vi "parse_add_vector_response.vi"(0 "headers":string, 5 "body":string, 11 "error in (no error)":errorcluster) -> (15 "error out":errorcluster)   [LabVIEW 2020, in "vector_weviate.lvclass"]
doc: "This VI parses the response of the Add Vector request"
uses:
  vector_weviate.lvclass
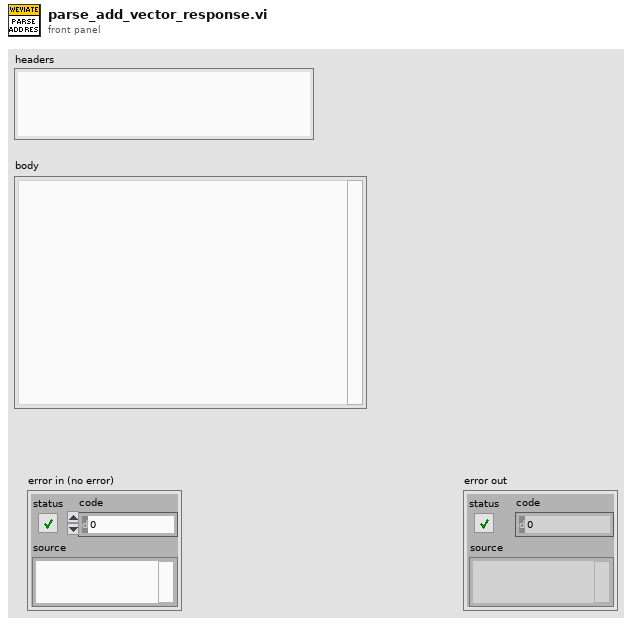
[diagram p1: front panel]
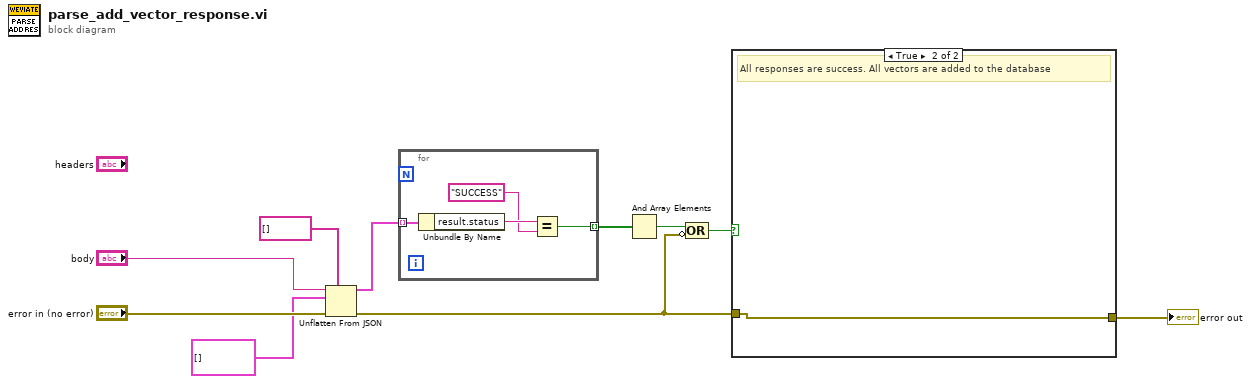
[diagram p0: block diagram]
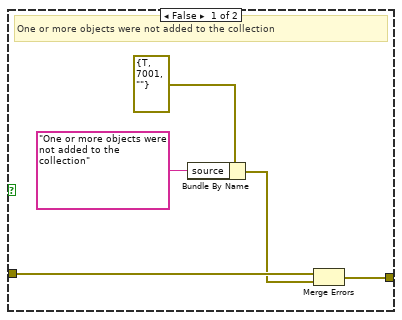
[diagram p2: hidden frame]
diagram:
  n1 = Unflatten From JSON(path=string[] [], JSON string="body", type and defaults=cluster{"result":cluster{"status":string}}[] [], error in (no error)="error in (no error)") -> (value=w6:cluster{"result":cluster{"status":string}}[], error out=w3:errorcluster)  [unwired: 3 in]
  n2 = for {
    tunnel: w6 -> [w14] mode=indexing
    tunnel: [w11] -> w5 mode=indexing
    n3 = Unbundle By Name(w14) -> ("result.status"=w13:string)
    n4 = Equal?(x=w13, y="SUCCESS") -> (x = y?=w11:bool)
  }
  n5 = And Array Elements(Boolean array=w5) -> (logical AND=w4:bool)
  n6 = Compound Arithmetic op=OR(w4, invert w3) -> (w2:bool)
  n7 = case shown="True" w2 {
    tunnel: w3 -> [w17 w20]
    tunnel: [w15 w20] -> w1
    frame False {
      # "One or more objects were not added to the collection"
      n8 = Bundle By Name(cluster=errorcluster {"status"=TRUE, "code"=7001, "source"=""} ("error constant"), "source"="One or more objects were not added to the collection" ("format string")) -> (w16:errorcluster)
      n9 = Merge Errors(w17, w16) -> (w15:errorcluster)
    }
    frame True {
      # "All responses are success. All vectors are added to the database"
    }
  }
  "error out" <- w1
